vi "GetLastnElemsfromArray.vi"(1 "array":dbl[][](array[numeric]), 2 "y":i32=40) -> (0 "deleted portion":dbl[][](array[numeric]))   [LabVIEW 2023]
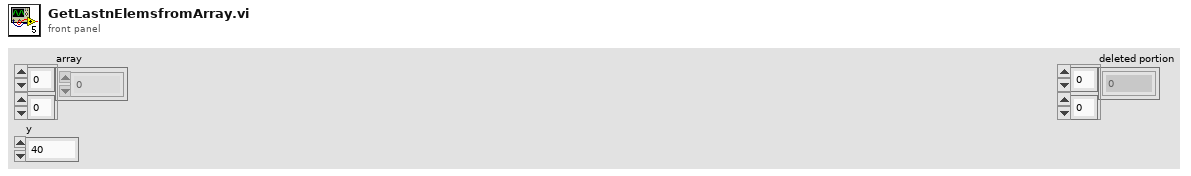
[diagram p1: front panel]
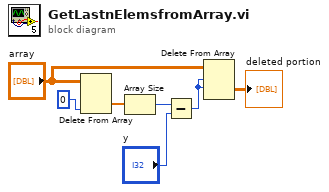
[diagram p0: block diagram]
diagram:
  n1 = Delete From Array(array="array", index (col)=0 ("disabled index (col)")) -> (deleted portion=w3:dbl[])  [unwired: 2 in, 1 out]
  n2 = Array Size(array=w3) -> (size(s)=w6:i32)
  n3 = Subtract(x=w6, y="y") -> (x-y=w4:i32)
  n4 = Delete From Array(array="array", length=w4, index (row)=w4) -> (deleted portion=→"deleted portion":dbl[][])  [unwired: 1 in, 1 out]
